vi "test.top.level.vi"() -> ()   [LabVIEW 2021]
uses:
  Test.Case.type.ctl
panel:
  out "All 512 Pass?":bool=TRUE
  out "All 256 Pass?":bool=TRUE
  out "Array 2":cluster{bool, bool}[](array[cluster])=[{TRUE, TRUE}, {TRUE, TRUE}, {TRUE, TRUE}, {TRUE, TRUE}, {TRUE, TRUE}, {TRUE, TRUE}, {TRUE, TRUE}, {TRUE, TRUE}, {TRUE, TRUE}, {TRUE, TRUE}, {TRUE, TRUE}, {TRUE, TRUE}, {TRUE, TRUE}, {TRUE, TRUE}, {TRUE, TRUE}, {TRUE, TRUE}, {TRUE, TRUE}, {TRUE, TRUE}, {TRUE, TRUE}, {TRUE, TRUE}, {TRUE, TRUE}, {TRUE, TRUE}, {TRUE, TRUE}, {TRUE, TRUE}, {TRUE, TRUE}, {TRUE, TRUE}, {TRUE, TRUE}, {TRUE, TRUE}, {TRUE, TRUE}, {TRUE, TRUE}, {TRUE, TRUE}, {TRUE, TRUE}, {TRUE, TRUE}, {TRUE, TRUE}, {TRUE, TRUE}, {TRUE, TRUE}, {TRUE, TRUE}, {TRUE, TRUE}, {TRUE, TRUE}, {TRUE, TRUE}, {TRUE, TRUE}, {TRUE, TRUE}, {TRUE, TRUE}, {TRUE, TRUE}, {TRUE, TRUE}, {TRUE, TRUE}, {TRUE, TRUE}, {TRUE, TRUE}, {TRUE, TRUE}, {TRUE, TRUE}, {TRUE, TRUE}, {TRUE, TRUE}, {TRUE, TRUE}, {TRUE, TRUE}, {TRUE, TRUE}, {TRUE, TRUE}, {TRUE, TRUE}, {TRUE, TRUE}, {TRUE, TRUE}, {TRUE, TRUE}, {TRUE, TRUE}, {TRUE, TRUE}, {TRUE, TRUE}, {TRUE, TRUE}, {TRUE, TRUE}, {TRUE, TRUE}, {TRUE, TRUE}, {TRUE, TRUE}, {TRUE, TRUE}, {TRUE, TRUE}, {TRUE, TRUE}, {TRUE, TRUE}, {TRUE, TRUE}, {TRUE, TRUE}, {TRUE, TRUE}, {TRUE, TRUE}, {TRUE, TRUE}, {TRUE, TRUE}, {TRUE, TRUE}, {TRUE, TRUE}, {TRUE, TRUE}, {TRUE, TRUE}, {TRUE, TRUE}, {TRUE, TRUE}, {TRUE, TRUE}, {TRUE, TRUE}, {TRUE, TRUE}, {TRUE, TRUE}, {TRUE, TRUE}, {TRUE, TRUE}, {TRUE, TRUE}, {TRUE, TRUE}, {TRUE, TRUE}, {TRUE, TRUE}, {TRUE, TRUE}, {TRUE, TRUE}, {TRUE, TRUE}, {TRUE, TRUE}, {TRUE, TRUE}, {TRUE, TRUE}, {TRUE, TRUE}, {TRUE, TRUE}, {TRUE, TRUE}, {TRUE, TRUE}, {TRUE, TRUE}, {TRUE, TRUE}, {TRUE, TRUE}, {TRUE, TRUE}, {TRUE, TRUE}, {TRUE, TRUE}, {TRUE, TRUE}, {TRUE, TRUE}, {TRUE, TRUE}, {TRUE, TRUE}, {TRUE, TRUE}, {TRUE, TRUE}, {TRUE, TRUE}, {TRUE, TRUE}, {TRUE, TRUE}, {TRUE, TRUE}, {TRUE, TRUE}, {TRUE, TRUE}, {TRUE, TRUE}, {TRUE, TRUE}, {TRUE, TRUE}, {TRUE, TRUE}, {TRUE, TRUE}, {TRUE, TRUE}, {TRUE, TRUE}, {TRUE, TRUE}, {TRUE, TRUE}, {TRUE, TRUE}, {TRUE, TRUE}, {TRUE, TRUE}, {TRUE, TRUE}, {TRUE, TRUE}, {TRUE, TRUE}, {TRUE, TRUE}, {TRUE, TRUE}, {TRUE, TRUE}, {TRUE, TRUE}, {TRUE, TRUE}, {TRUE, TRUE}, {TRUE, TRUE}, {TRUE, TRUE}, {TRUE, TRUE}, {TRUE, TRUE}, {TRUE, TRUE}, {TRUE, TRUE}, {TRUE, TRUE}, {TRUE, TRUE}, {TRUE, TRUE}, {TRUE, TRUE}, {TRUE, TRUE}, {TRUE, TRUE}, {TRUE, TRUE}, {TRUE, TRUE}, {TRUE, TRUE}, {TRUE, TRUE}, {TRUE, TRUE}, {TRUE, TRUE}, {TRUE, TRUE}, {TRUE, TRUE}, {TRUE, TRUE}, {TRUE, TRUE}, {TRUE, TRUE}, {TRUE, TRUE}]
  out "Array":u8[](array[numeric])=[65, 115, 32, 69, 115, 116, 104, 97, 32, 115, 116, 105, 114, 114, 101, 100, 32, 116, 104, 101, 32, 116, 104, 105, 99, 107, 32, 106, 97, 109, 32, 104, 101, 32, 116, 104, 111, 117, 103, 104, 116, 32, 84, 119, 111, 32, 84, 104, 111, 117, 103, 104, 116, 115, 32, 97, 110, 100, 32, 116, 104, 101, 32, 84, 119, 111, 32, 84, 104, 111, 117, 103, 104, 116, 115, 32, 104, 101, 32, 116, 104, 111, 117, 103, 104, 116, 32, 119, 101, 114, 101, 32, 116, 104, 101, 115, 101, 58, 32, 97, 41, 32, 65, 110, 121, 116, 104, 105, 110, 103, 32, 99, 97, 110, 32, 104, 97, 112, 112, 101, 110, 32, 116, 111, 32, 97, 110, 121, 111, 110, 101, 46, 32, 97, 110, 100, 32, 98, 41, 32, 73, 116, 32, 105, 115, 32, 98, 101, 115, 116, 32, 116, 111, 32, 98, 101, 32, 112, 114, 101, 112, 97, 114, 101, 100, 46] format="%.0x"
  out "512 matches?":bool=TRUE
  out "Final.State 512":u64[](array[numeric])=[13301219531156492385, 11127854853417562052, 524277580094970210, 1540142370391429374, 12412996341010901443, 3598767773402858399, 924216014969962459, 18423737124033093736, 9041965587285169724, 11946436709797590620, 9598377346200053498, 15609136642136624313, 13839031544369048776, 16785932279372823442, 18077763469661243185, 6037779733261654142, 5492308379086555739, 2813253888995526086, 3560799791317313623, 11061351188809493633, 14966076467780343448, 9073521057931985780, 7504373216799846216, 2649547696616143726, 14741899879960970636] format="%.0x"
  out "256 matches?":bool=TRUE
  out "Final.State 256":u64[](array[numeric])=[11676268880411235193, 13451318828874210226, 4095211424469938024, 15068679232636183629, 7753535997560901512, 5388403742991398886, 18434487315843317224, 9964010514430008916, 15544274158139793918, 17249301923950297777, 11191994372900048372, 9929105044359600294, 9415787041053954757, 3504658296181967959, 5125580019117546070, 12884011986622445834, 10134502102761320058, 17607174279953371043, 17308940434400663160, 5579560056542968276, 9133654056512198443, 18102584358251476685, 2528813078336136997, 14545830983934253368, 1290234347948013036] format="%.0x"
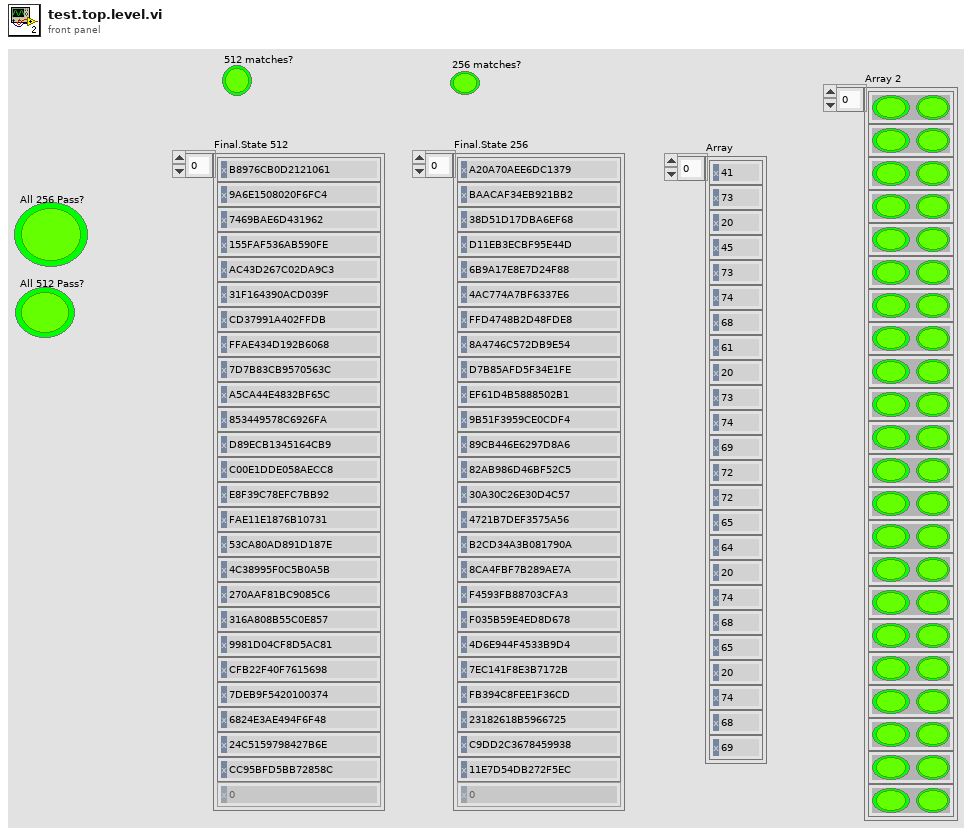
[diagram p1: front panel]
types:
  T1 = typedef "Test.Case.type.ctl" = cluster{"input_size":i32, "expected_hash256":string, "expected_hash512":string}
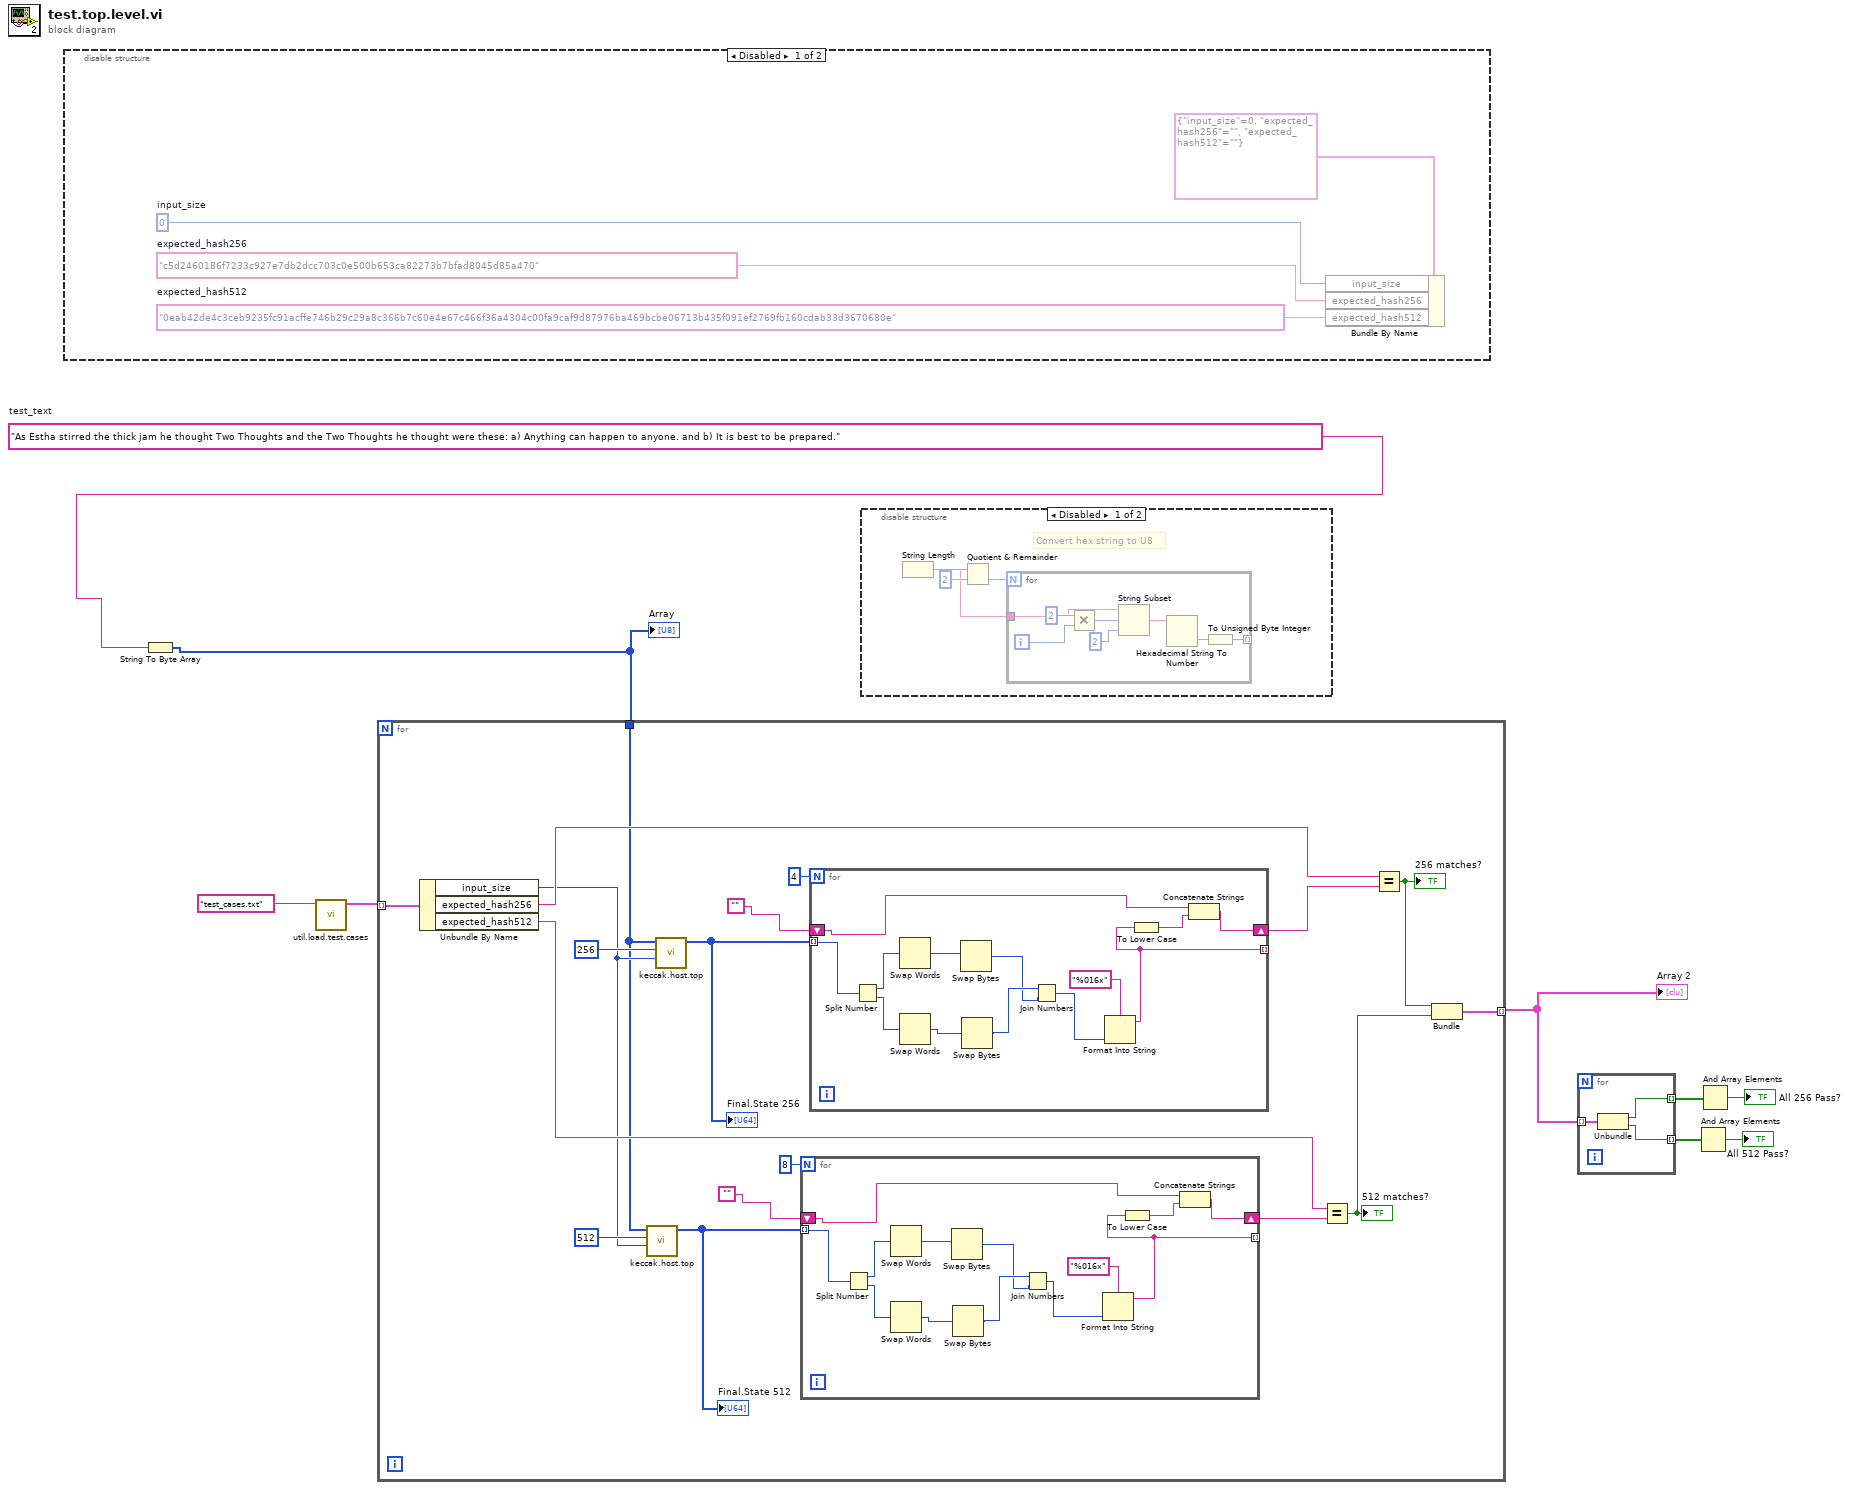
[diagram p0: block diagram]
diagram:
  w7 = "As Estha stirred the thick jam he thought Two Thoughts and the Two Thoughts he thought were these: a) Anything can happen to anyone. and b) It is best to be prepared."  # test_text
  n1 = disable-structure shown="Disabled" {
    frame Disabled {
      w12 = "0eab42de4c3ceb9235fc91acffe746b29c29a8c366b7c60e4e67c466f36a4304c00fa9caf9d87976ba469bcbe06713b435f091ef2769fb160cdab33d3670680e"  # expected_hash512
      w11 = "c5d2460186f7233c927e7db2dcc703c0e500b653ca82273b7bfad8045d85a470"  # expected_hash256
      w10 = 0  # input_size
      n2 = Bundle By Name(cluster=T1 {"input_size"=0, "expected_hash256"="", "expected_hash512"=""}, "input_size"=w10, "expected_hash256"=w11, "expected_hash512"=w12) -> ()  [unwired: 1 out]
    }
    frame Enabled {
    }
  }
  n3 = String To Byte Array(string=w7) -> (unsigned byte array=w6:u8[])
  "Array" <- w6
  n4 = call "util.load.test.cases.vi"("String"="test_cases.txt") -> ("Array"=w8:T1[])  [unwired: 10 in]
  n5 = for {
    tunnel: w8 -> [w19] mode=indexing
    tunnel: w6 -> [w17]
    tunnel: [w14] -> w5 mode=indexing
    n6 = Unbundle By Name(w19) -> ("input_size"=w18:i32, "expected_hash256"=w26:string, "expected_hash512"=w20:string)
    n7 = call "keccak.host.top.vi"("size"=w18, "Bits.in"=512, "Data.in"=w17) -> ("Final.State"=w25:u64[])  [unwired: 8 in]
    "Final.State 512" <- w25
    n8 = call "keccak.host.top.vi"("size"=w18, "Bits.in"=256, "Data.in"=w17) -> ("Final.State"=w31:u64[])  [unwired: 8 in]
    "Final.State 256" <- w31
    n9 = for {
      N: 8 -> [_]
      tunnel: w25 -> [w44] mode=indexing
      tunnel: [w32] -> _ mode=indexing
      shift-right: [w37] -> w21
      shift-left: "" -> [w36]
      n10 = Split Number(x=w44) -> (hi(x)=w43:u32, lo(x)=w42:u32)
      n11 = Swap Words(1:w43) -> (0:w41:u32)
      n12 = Swap Words(1:w42) -> (0:w40:u32)
      n13 = Swap Bytes(anything=w41) -> (byte swapped=w38:u32)
      n14 = Swap Bytes(anything=w40) -> (byte swapped=w39:u32)
      n15 = Join Numbers(hi=w39, lo=w38) -> ((hi.lo)=w34:u64)
      n16 = Format Into String(format string="%016x", w34) -> (resulting string=w32:string)  [unwired: 2 in, 1 out]
      n17 = To Lower Case(string=w32) -> (all lower case string=w35:string)
      n18 = Concatenate Strings(w36, w35) -> (w37:string)
    }
    n19 = for {
      N: 4 -> [_]
      tunnel: w31 -> [w57] mode=indexing
      tunnel: [w45] -> _ mode=indexing
      shift-right: [w50] -> w28
      shift-left: "" -> [w49]
      n20 = Split Number(x=w57) -> (hi(x)=w56:u32, lo(x)=w55:u32)
      n21 = Swap Words(1:w56) -> (0:w54:u32)
      n22 = Swap Words(1:w55) -> (0:w53:u32)
      n23 = Swap Bytes(anything=w54) -> (byte swapped=w51:u32)
      n24 = Swap Bytes(anything=w53) -> (byte swapped=w52:u32)
      n25 = Join Numbers(hi=w52, lo=w51) -> ((hi.lo)=w47:u64)
      n26 = Format Into String(format string="%016x", w47) -> (resulting string=w45:string)  [unwired: 2 in, 1 out]
      n27 = To Lower Case(string=w45) -> (all lower case string=w48:string)
      n28 = Concatenate Strings(w49, w48) -> (w50:string)
    }
    n29 = Equal?(x=w20, y=w21) -> (x = y?=w15:bool)
    "512 matches?" <- w15
    n30 = Equal?(x=w26, y=w28) -> (x = y?=w16:bool)
    "256 matches?" <- w16
    n31 = Bundle(w16, w15) -> (w14:cluster{bool, bool})  [unwired: 1 in]
  }
  "Array 2" <- w5
  n32 = disable-structure shown="Disabled" {
    frame Disabled {
      # "Convert hex string to U8"
      n33 = String Length() -> (string=w58:string, length=w61:i32)
      n34 = Quotient & Remainder(x=w61, y=2) -> (floor(x/y)=w59:i32)  [unwired: 1 out]
      n35 = for {
        N: w59 -> [_]
        tunnel: w58 -> [w65]
        tunnel: [w62] -> _ mode=indexing
        i -> [w69]
        n36 = Multiply(x=2, y=w69) -> (x*y=w68:i32)
        n37 = String Subset(string=w65, offset (0)=w68, length (rest)=2 ("length (rest)")) -> (substring=w64:string)
        n38 = Hexadecimal String To Number(string=w64) -> (number=w63:u32)  [unwired: 2 in, 1 out]
        n39 = To Unsigned Byte Integer(number=w63) -> (unsigned 8bit integer=w62:u8)
      }
    }
    frame Enabled {
    }
  }
  n40 = for {
    tunnel: w5 -> [w72] mode=indexing
    tunnel: [w71] -> w4 mode=indexing
    tunnel: [w70] -> w3 mode=indexing
    n41 = Unbundle(w72) -> (w71:bool, w70:bool)
  }
  n42 = And Array Elements(Boolean array=w3) -> (logical AND=→"All 512 Pass?":bool)
  n43 = And Array Elements(Boolean array=w4) -> (logical AND=→"All 256 Pass?":bool)
